vi "GetGlobalVariable.vi"   [LabVIEW 2018, in "Aerotech.lvlib"]
uses:
  Aerotech.lvlib
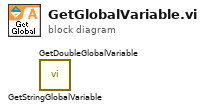
[diagram p0: block diagram]
diagram:
  n1 = call "GetStringGlobalVariable.vi"() -> ()  [unwired: 9 in, 3 out]
  n2 = call "GetDoubleGlobalVariable.vi"() -> ()  [unwired: 9 in, 3 out]
